vi "MOSES Background 4_v8.vi"(5 "Array Input":refnum<vi>) -> (0 "PSU":dbl[](graph), 1 "Values to Output":T1, 2 "Power Supply Filter Input":dbl[](graph), 3 "ROE":dbl[](graph))   [LabVIEW 2013]
uses:
  Instance           9 26Saved   MOSES Background 4 .vi
  Instance          14 26Saved   MOSES Background 4 .vi
  Instance           8 26Saved   MOSES Background 4 .vi
  Instance          21 26Saved   MOSES Background 4 .vi
  Instance           3 26Saved   MOSES Background 4 .vi
  Instance          22 26Saved   MOSES Background 4 .vi
  Instance           6 26Saved   MOSES Background 4 .vi
  Instance          23 26Saved   MOSES Background 4 .vi
  Instance           7 26Saved   MOSES Background 4 .vi
  Instance          24 26Saved   MOSES Background 4 .vi
  Instance           5 26Saved   MOSES Background 4 .vi
  Instance          15 26Saved   MOSES Background 4 .vi
  Instance           4 26Saved   MOSES Background 4 .vi
  Instance          16 26Saved   MOSES Background 4 .vi
  Instance          28 26Saved   MOSES Background 4 .vi
  Instance          17 26Saved   MOSES Background 4 .vi
  Instance           2 26Saved   MOSES Background 4 .vi
  Instance          18 26Saved   MOSES Background 4 .vi
  Instance           1 26Saved   MOSES Background 4 .vi
  Instance          19 26Saved   MOSES Background 4 .vi
  Instance          12 26Saved   MOSES Background 4 .vi
  Instance          20 26Saved   MOSES Background 4 .vi
  Instance          10 26Saved   MOSES Background 4 .vi
  Instance          26 26Saved   MOSES Background 4 .vi
  Instance          11 26Saved   MOSES Background 4 .vi
  Instance          25 26Saved   MOSES Background 4 .vi
  Instance          13 26Saved   MOSES Background 4 .vi
  Instance          27 26Saved   MOSES Background 4 .vi
panel:
  out "Boolean 17":bool
  out "Boolean 16":bool
  out "Boolean 15":bool
  out "Boolean 14":bool
  out "Boolean 13":bool
  out "Boolean 41":bool
  out "Boolean 40":bool
  out "Boolean 39":bool
  out "Boolean 38":bool
  out "Boolean 37":bool
  out "Boolean 36":bool
  out "Boolean 35":bool
  out "Boolean 34":bool
  out "Boolean 33":bool
  out "Boolean 32":bool
  out "Boolean 12":bool
  out "Boolean 11":bool
  out "Boolean 10":bool
  out "Boolean 84":bool
  out "Boolean 83":bool
  out "T_PSU, PSU Temp.":dbl
  out "Boolean 82":bool
  out "Boolean 81":bool
  out "T_ROE, ROE Temp.":dbl
  in  "stop 4":bool
  out "ROE_PSI, ROE power supply input current":dbl
  out "ROE_PSV, ROE power supply input voltage":dbl
  out "I_pf5, Premod filter 5V input current":dbl
  out "HAFI, H-alpha filter current":dbl
  out "S28I, Shutter 28V power current":dbl
  out "Ipf12+, Premod filter positive 12V input current":dbl
  out "If_in":dbl[](graph)
  out "Boolean 31":bool
  out "Boolean 30":bool
  out "Boolean 29":bool
  out "If_in, Power supply filter input current":dbl
  out "Boolean 23":bool
  out "Boolean 22":bool
  out "Boolean 9":bool
  out "Boolean 8":bool
  out "Boolean 7":bool
  out "HACV, H-alpha camera voltage":dbl
  out "HAFV, H-alpha filter voltage":dbl
  out "Boolean 21":bool
  out "Boolean 20":bool
  out "Boolean 19":bool
  out "Boolean 18":bool
  out "S28V, Shutter 28V power voltage":dbl
  out "T5V, Thermal 5V power voltage":dbl
  out "V5s, MGA2805S output voltage":dbl
  out "Vina_0y":dbl
  out "Vina_-y":dbl
  out "Vina_+y, INA330 Output":dbl
  out "Vex_0y":dbl
  out "Vex_-y":dbl
  out "Vex_+y":dbl
  out "Va_0y":dbl
  out "Va_-y":dbl
  out "Waveform Chart 2":dbl[](graph)
  out "Va_+y, Thermistor Voltage":dbl
  # "A"
  # "A"
  # "V"
  # "mA"
  # "C"
  # "C"
  # "V"
  # "V"
  # "V"
  # "V"
  # "V"
  # "A"
  # "mA"
  # "mA"
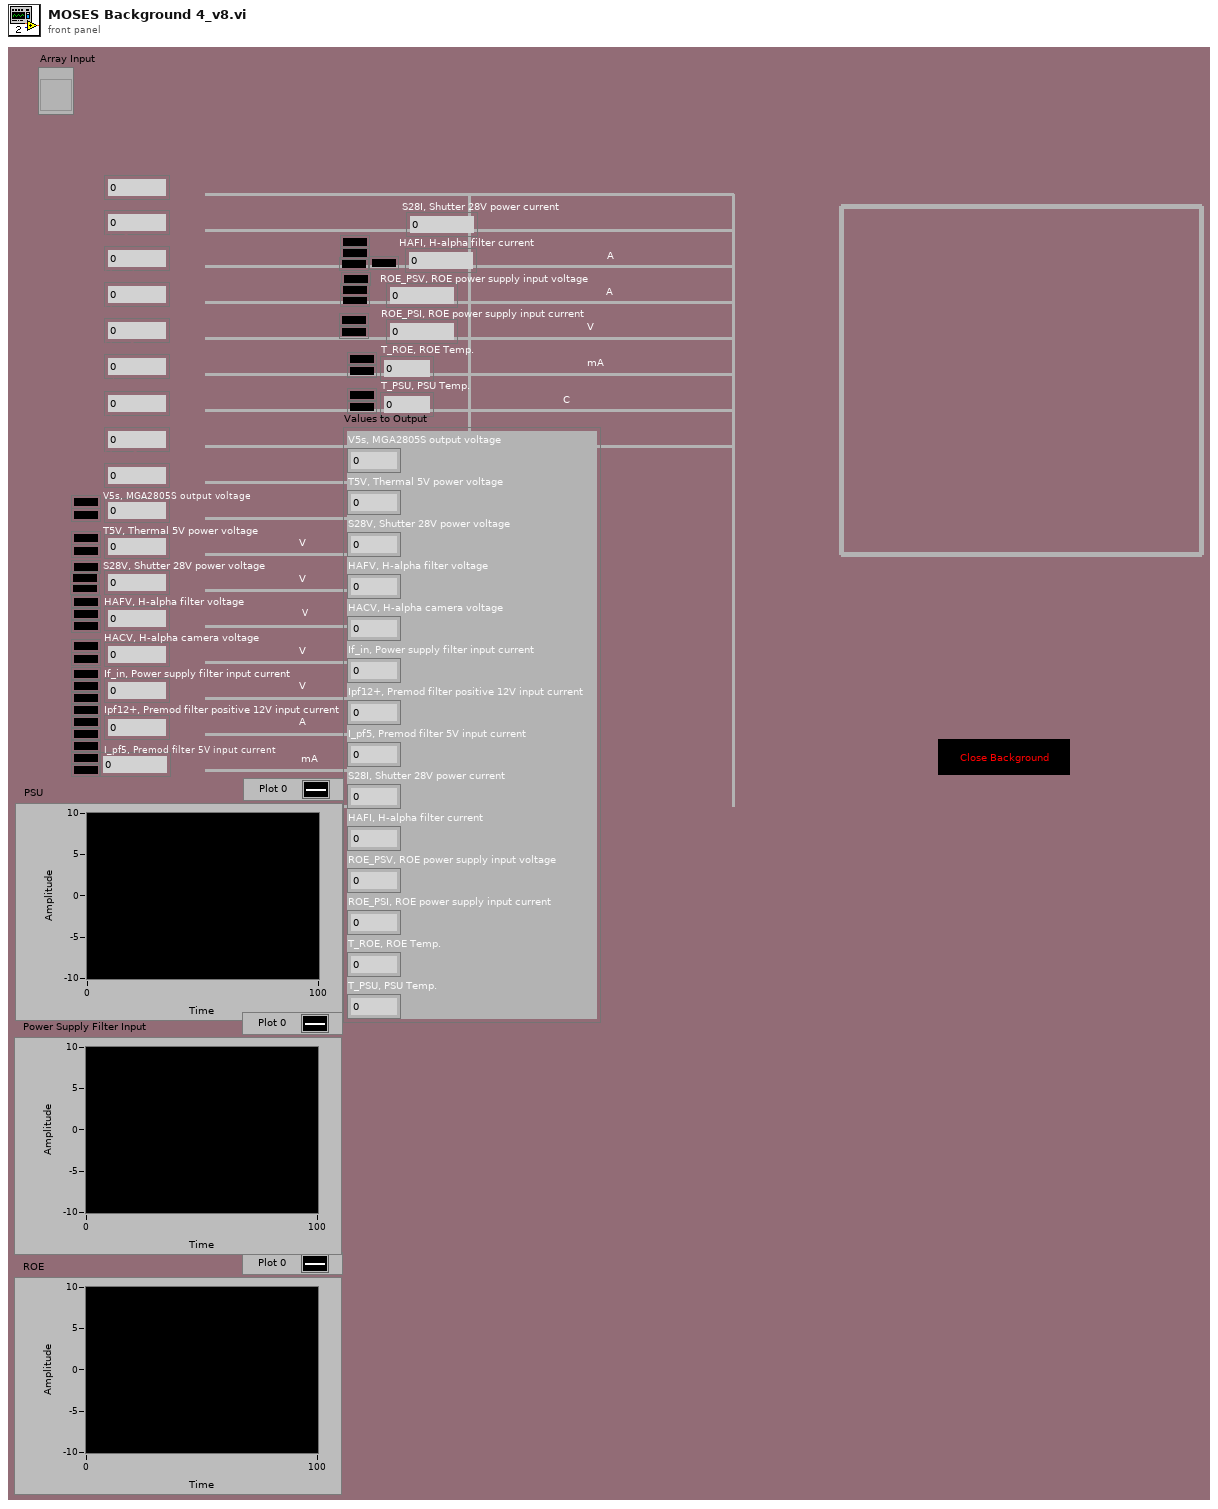
[diagram p1: front panel]
types:
  T1 = cluster{"V5s, MGA2805S output voltage":dbl, "T5V, Thermal 5V power voltage":dbl, "S28V, Shutter 28V power voltage":dbl, "HAFV, H-alpha filter voltage":dbl, "HACV, H-alpha camera voltage":dbl, "If_in, Power supply filter input current":dbl, "Ipf12+, Premod filter positive 12V input current":dbl, "I_pf5, Premod filter 5V input current":dbl, "S28I, Shutter 28V power current":dbl, "HAFI, H-alpha filter current":dbl, "ROE_PSV, ROE power supply input voltage":dbl, "ROE_PSI, ROE power supply input current":dbl, "T_ROE, ROE Temp.":dbl, "T_PSU, PSU Temp.":dbl}
  T2 = cluster{"Value[0]":dbl, "Value[1]":dbl, "Value[2]":dbl, "Value[3]":dbl, "Value[4]":dbl, "Value[5]":dbl, "Value[6]":dbl, "Value[7]":dbl, "Value[8]":dbl, "Value[9]":dbl, "Value[10]":dbl, "Value[11]":dbl, "Value[12]":dbl, "Value[13]":dbl, "Value[14]":dbl, "Value[15]":dbl, "Value[16]":dbl, "Value[17]":dbl, "Value[18]":dbl, "Value[19]":dbl, "Value[20]":dbl, "Value[21]":dbl, "Value[22]":dbl, "Value[23]":dbl, "Value[24]":dbl, "Value[25]":dbl, "Value[26]":dbl, "Value[27]":dbl, "Value[28]":dbl, "Value[29]":dbl, "Value[30]":dbl, "Value[31]":dbl, "Value[32]":dbl, "Value[33]":dbl, "Value[34]":dbl, "Value[35]":dbl, "Value[36]":dbl, "Value[37]":dbl, "Value[38]":dbl, "Value[39]":dbl, "Value[40]":dbl, "Value[41]":dbl, "Value[42]":dbl, "Value[43]":dbl, "Value[44]":dbl, "Value[45]":dbl, "Value[46]":dbl, "Value[47]":dbl, "Value[48]":dbl, "Value[49]":dbl, "Value[50]":dbl, "Value[51]":dbl, "Value[52]":dbl, "Value[53]":dbl, "Value[54]":dbl, "Value[55]":dbl, "Value[56]":dbl, "Value[57]":dbl, "Value[58]":dbl, "Value[59]":dbl, "Value[60]":dbl, "Value[61]":dbl, "Value[62]":dbl, "Value[63]":dbl, "Value[64]":dbl, "Value[65]":dbl, "Value[66]":dbl, "Value[67]":dbl, "Value[68]":dbl, "Value[69]":dbl}
  T3 = cluster{"[0]":dbl, "[1]":dbl, "[2]":dbl, "[3]":dbl, "[4]":dbl, "[5]":dbl, "[6]":dbl, "[7]":dbl, "[8]":dbl, "[9]":dbl, "[10]":dbl, "[11]":dbl, "[12]":dbl, "[13]":dbl}
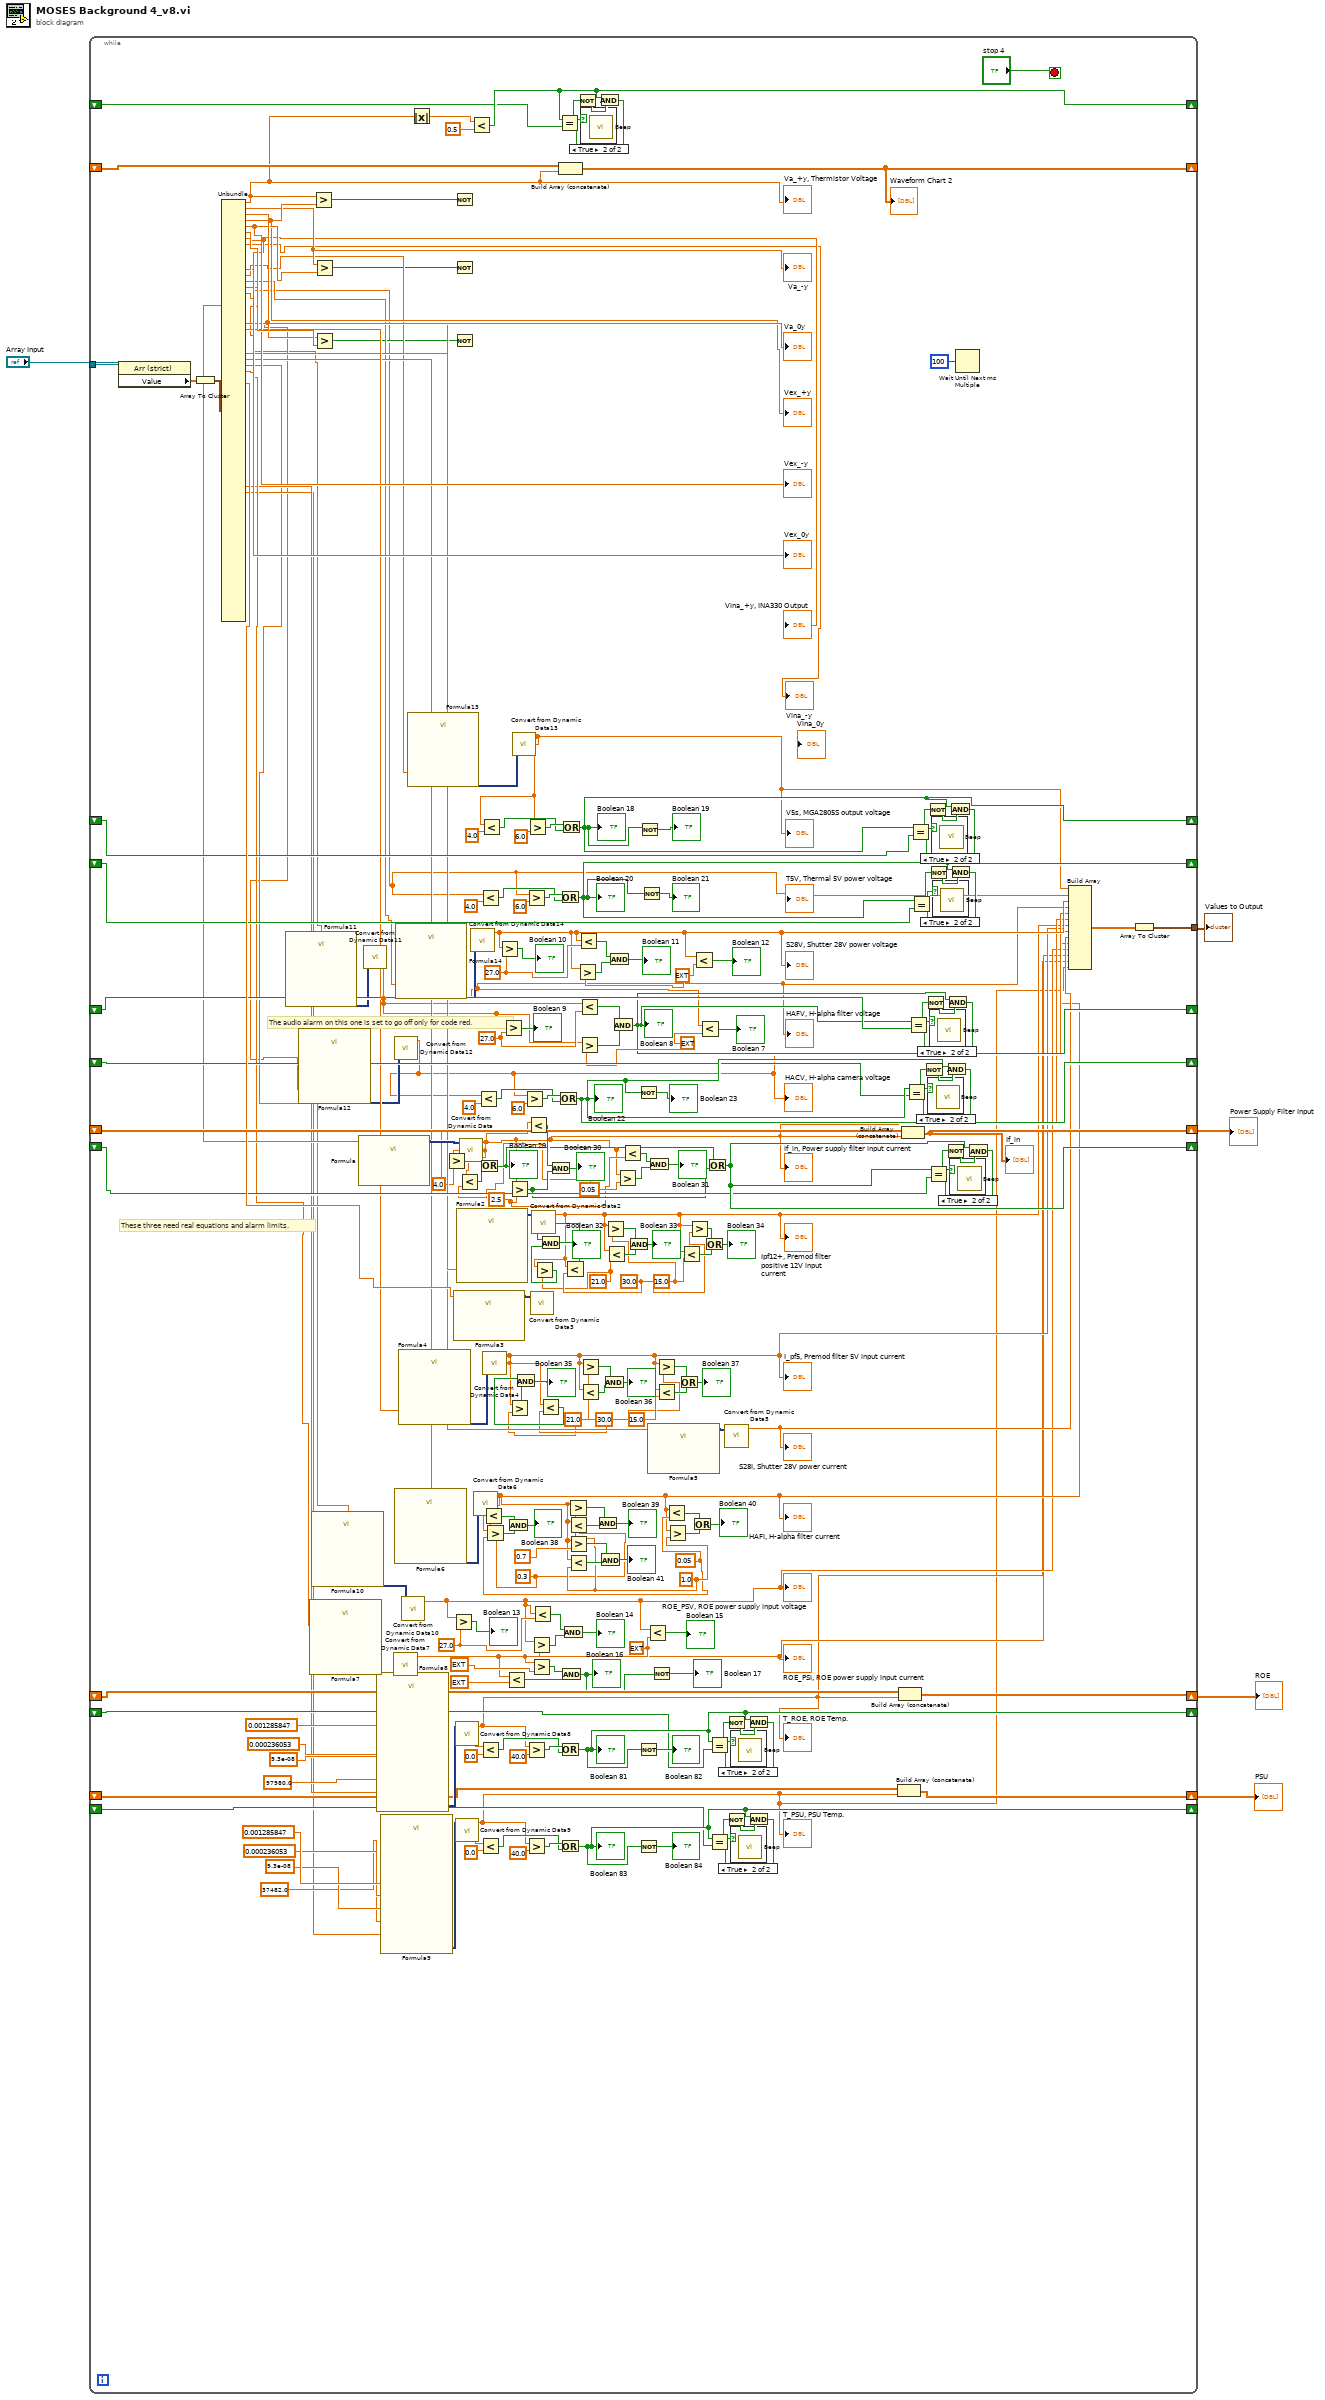
[diagram p0: block diagram]
diagram:
  n1 = while {
    tunnel: "Array Input" -> [w226]
    shift-right: [w222] -> _
    shift-left: _ -> [w223]
    shift-right: [w198] -> w1
    shift-left: _ -> [w199]
    shift-right: [w180] -> _
    shift-left: _ -> [w179]
    shift-right: [w163] -> _
    shift-left: _ -> [w162]
    shift-right: [w96] -> _
    shift-left: _ -> [w161]
    shift-right: [w160] -> _
    shift-left: _ -> [w159]
    shift-right: [w158] -> _
    shift-left: _ -> [w157]
    shift-right: [w156] -> _
    shift-left: _ -> [w155]
    shift-right: [w135] -> _
    shift-left: _ -> [w134]
    shift-right: [w133] -> _
    shift-left: _ -> [w132]
    shift-right: [w129] -> w3
    shift-left: _ -> [w131]
    shift-right: [w128] -> w2
    shift-left: _ -> [w130]
    tunnel: [w6] -> w4
    stop <- "stop 4" stop-if-true
    w42 = 27.0 ("y")
    w37 = ext 20.0 ("y")
    w45 = 0.05 ("y")
    w44 = 0.3 ("y")
    w46 = 1.0 ("y")
    w62 = 15.0 ("y")
    w61 = 30.0 ("y")
    w60 = 21.0 ("y")
    w73 = 15.0 ("y")
    w72 = 30.0 ("y")
    w22 = 21.0 ("y")
    w94 = 27.0 ("y")
    w90 = ext 20.0 ("y")
    w27 = 0.05 ("y")
    w85 = 4.0 ("y")
    w23 = 2.5 ("y")
    w99 = ext 20.0 ("y")
    w206 = 27.0 ("y")
    # "These three need real equations and alarm limits."
    # "The audio alarm on this one is set to go off only for code red."
    n2 = property class="Arr (strict)"(reference=w226) -> ("Value"=w225:dbl[])  [unwired: 1 in, 2 out]
    n3 = Array To Cluster(array=w225) -> (cluster=w224:T2)
    n4 = Unbundle(w224) -> ("Value[0]"=w186:dbl, "Value[1]"=w187:dbl, "Value[2]"=w220:dbl, "Value[3]"=w188:dbl, "Value[4]"=w219:dbl, "Value[5]"=w221:dbl, "Value[6]"=→"Vex_0y" →"Vina_+y, INA330 Output":dbl, "Value[7]"=→"Vina_-y":dbl, "Value[11]"=w102:dbl, "Value[12]"=w20:dbl, "Value[13]"=w100:dbl, "Value[14]"=w104:dbl, "Value[15]"=w106:dbl, "Value[17]"=w125:dbl, "Value[20]"=w124:dbl, "Value[21]"=w123:dbl, "Value[25]"=w122:dbl, "Value[26]"=w121:dbl, "Value[27]"=w108:dbl, "Value[28]"=w120:dbl, "Value[30]"=w195:dbl, "Value[47]"=w111:dbl, "Value[48]"=w110:dbl)  [unwired: 47 out]
    "Va_+y, Thermistor Voltage" <- w186
    "Va_-y" <- w187
    "Va_0y" <- w220
    "Vex_+y" <- w188
    "Vex_-y" <- w219
    "T5V, Thermal 5V power voltage" <- w20
    n5 = call "Formula11"("X1"=w104) -> ("Result"=w105:dynamicdata)  [unwired: 13 in, 1 out]
    n6 = call "Formula12"("X1"=w106) -> ("Result"=w107:dynamicdata)  [unwired: 13 in, 1 out]
    n7 = call "Formula7"("X1"=w120) -> ("Result"=w191:dynamicdata)  [unwired: 13 in, 1 out]
    n8 = Greater?(x=w186, y=w188) -> (0:w190:bool)
    n9 = call "Formula10"("X1"=w108) -> ("Result"=w109:dynamicdata)  [unwired: 13 in, 1 out]
    n10 = Greater?(x=w187, y=w219) -> (0:w84:bool)
    n11 = Greater?(x=w220, y=w221) -> (0:w83:bool)
    n12 = call "Formula"("X1"=w125) -> ("Result"=w200:dynamicdata)  [unwired: 13 in, 1 out]
    n13 = call "Convert from Dynamic Data11"("Dynamic Data Type"=w105) -> ("Scalar"=w18:dbl)  [unwired: 3 in]
    "HAFV, H-alpha filter voltage" <- w18
    n14 = call "Formula8"("a"=0.001285847 ("double precision float"), "v0"=w111, "b"=0.000236053 ("double precision float"), "c"=9.3e-08 ("double precision float"), "R"=97980.0 ("double precision float")) -> ("Result"=w148:dynamicdata)  [unwired: 9 in, 1 out]
    n15 = call "Formula9"("a"=0.001285847 ("double precision float"), "v0"=w110, "b"=0.000236053 ("double precision float"), "c"=9.3e-08 ("double precision float"), "R"=37482.0 ("double precision float")) -> ("Result"=w139:dynamicdata)  [unwired: 9 in, 1 out]
    n16 = call "Convert from Dynamic Data7"("Dynamic Data Type"=w191) -> ("Scalar"=w10:dbl)  [unwired: 3 in]
    "ROE_PSI, ROE power supply input current" <- w10
    n17 = call "Convert from Dynamic Data12"("Dynamic Data Type"=w107) -> ("Scalar"=w17:dbl)  [unwired: 3 in]
    "HACV, H-alpha camera voltage" <- w17
    n18 = call "Formula6"("X1"=w121) -> ("Result"=w192:dynamicdata)  [unwired: 13 in, 1 out]
    n19 = call "Formula14"("X1"=w100) -> ("Result"=w101:dynamicdata)  [unwired: 13 in, 1 out]
    n20 = call "Formula4"("X1"=w123) -> ("Result"=w194:dynamicdata)  [unwired: 13 in, 1 out]
    n21 = call "Convert from Dynamic Data10"("Dynamic Data Type"=w109) -> ("Scalar"=w11:dbl)  [unwired: 3 in]
    "ROE_PSV, ROE power supply input voltage" <- w11
    n22 = call "Formula13"("X1"=w102) -> ("Result"=w103:dynamicdata)  [unwired: 13 in, 1 out]
    n23 = Absolute Value(x=w186) -> (abs(x)=w184:dbl)
    n24 = Greater?(x=w11, y=w42) -> (0:→"Boolean 13":bool)
    n25 = Not(x=w190) -> ()  [unwired: 1 out]
    n26 = Not(x=w84) -> ()  [unwired: 1 out]
    n27 = Not(x=w83) -> ()  [unwired: 1 out]
    n28 = call "Formula3"("X1"=w195) -> ("Result"=w196:dynamicdata)  [unwired: 13 in, 1 out]
    n29 = call "Convert from Dynamic Data8"("Dynamic Data Type"=w148) -> ("Scalar"=w9:dbl)  [unwired: 3 in]
    "T_ROE, ROE Temp." <- w9
    n30 = call "Convert from Dynamic Data9"("Dynamic Data Type"=w139) -> ("Scalar"=w8:dbl)  [unwired: 3 in]
    "T_PSU, PSU Temp." <- w8
    n31 = call "Formula2"("X1"=w124) -> ("Result"=w197:dynamicdata)  [unwired: 13 in, 1 out]
    n32 = call "Convert from Dynamic Data"("Dynamic Data Type"=w200) -> ("Scalar"=w16:dbl)  [unwired: 3 in]
    "If_in, Power supply filter input current" <- w16
    n33 = Greater?(x=w16, y=w85) -> (0:w28:bool)
    n34 = Less?(x=w16, y=w27) -> (x < y?=w30:bool)
    n35 = Less?(x=w184, y=0.5) -> (x < y?=w180:bool)
    n36 = call "Convert from Dynamic Data14"("Dynamic Data Type"=w101) -> ("Scalar"=w19:dbl)  [unwired: 3 in]
    "S28V, Shutter 28V power voltage" <- w19
    n37 = call "Convert from Dynamic Data6"("Dynamic Data Type"=w192) -> ("Scalar"=w12:dbl)  [unwired: 3 in]
    "HAFI, H-alpha filter current" <- w12
    n38 = Less?(x=w17, y=4.0) -> (x < y?=w202:bool)
    n39 = Or(x=w28, y=w30) -> (x .or. y?=w29:bool)
    "Boolean 29" <- w29
    n40 = Less?(x=w20, y=4.0) -> (x < y?=w210:bool)
    n41 = Less?(x=w9, y=0.0) -> (x < y?=w150:bool)
    n42 = Less?(x=w8, y=0.0) -> (x < y?=w141:bool)
    n43 = Less?(x=w12, y=w44) -> (x < y?=w58:bool)
    n44 = call "Convert from Dynamic Data4"("Dynamic Data Type"=w194) -> ("Scalar"=w14:dbl)  [unwired: 3 in]
    "I_pf5, Premod filter 5V input current" <- w14
    n45 = Greater?(x=w12, y=w45) -> (0:w59:bool)
    n46 = Greater?(x=w19, y=w94) -> (0:→"Boolean 10":bool)
    n47 = Greater?(x=w18, y=w206) -> (0:→"Boolean 9":bool)
    n48 = Less?(x=w10, y=ext 390.0) -> (x < y?=w34:bool)
    n49 = And(x=w58, y=w59) -> (x .and. y?=→"Boolean 38":bool)
    n50 = Greater?(x=w16, y=w23) -> (0:w88:bool)
    n51 = Greater?(x=w14, y=w60) -> (0:w71:bool)
    n52 = call "Convert from Dynamic Data13"("Dynamic Data Type"=w103) -> ("Scalar"=w21:dbl)  [unwired: 3 in]
    "V5s, MGA2805S output voltage" <- w21
    n53 = Less?(x=w21, y=4.0) -> (x < y?=w215:bool)
    n54 = Greater?(x=w17, y=6.0) -> (0:w203:bool)
    n55 = Greater?(x=w20, y=6.0) -> (0:w211:bool)
    n56 = Greater?(x=w9, y=40.0) -> (0:w151:bool)
    n57 = Greater?(x=w8, y=40.0) -> (0:w142:bool)
    n58 = Greater?(x=w21, y=6.0) -> (0:w216:bool)
    n59 = Less?(x=w16, y=w85) -> (x < y?=w86:bool)
    n60 = Greater?(x=w10, y=ext 250.0) -> (0:w33:bool)
    n61 = call "Convert from Dynamic Data3"("Dynamic Data Type"=w196) -> ()  [unwired: 3 in, 1 out]
    n62 = Greater?(x=w11, y=w37) -> (0:w41:bool)
    n63 = Less?(x=w11, y=w42) -> (x < y?=w40:bool)
    n64 = call "Convert from Dynamic Data2"("Dynamic Data Type"=w197) -> ("Scalar"=w15:dbl)  [unwired: 3 in]
    "Ipf12+, Premod filter positive 12V input current" <- w15
    n65 = Greater?(x=w15, y=w22) -> (0:w82:bool)
    n66 = Less?(x=w14, y=w61) -> (x < y?=w70:bool)
    n67 = And(x=w70, y=w71) -> (x .and. y?=→"Boolean 35":bool)
    n68 = And(x=w86, y=w88) -> (x .and. y?=→"Boolean 30":bool)
    n69 = Or(x=w203, y=w202) -> (x .or. y?=w163:bool)
    "Boolean 22" <- w163
    n70 = Equal?(x=w180, y=w179) -> (x = y?=w181:bool)
    n71 = Build Array (concatenate)(w223, w186) -> (w222:dbl[])
    "Waveform Chart 2" <- w222
    n72 = Or(x=w211, y=w210) -> (x .or. y?=w160:bool)
    "Boolean 20" <- w160
    n73 = Or(x=w151, y=w150) -> (x .or. y?=w135:bool)
    "Boolean 81" <- w135
    n74 = Or(x=w142, y=w141) -> (x .or. y?=w133:bool)
    "Boolean 83" <- w133
    n75 = Or(x=w216, y=w215) -> (x .or. y?=w158:bool)
    "Boolean 18" <- w158
    n76 = And(x=w33, y=w34) -> (x .and. y?=w32:bool)
    "Boolean 16" <- w32
    n77 = And(x=w40, y=w41) -> (x .and. y?=→"Boolean 14":bool)
    n78 = Less?(x=w15, y=w72) -> (x < y?=w81:bool)
    n79 = And(x=w81, y=w82) -> (x .and. y?=→"Boolean 32":bool)
    n80 = Greater?(x=w12, y=w44) -> (0:w56:bool)
    n81 = Less?(x=w12, y=w46) -> (x < y?=w55:bool)
    n82 = Greater?(x=w12, y=0.7) -> (0:w52:bool)
    n83 = Less?(x=w12, y=w46) -> (x < y?=w53:bool)
    n84 = Not(x=w181) -> (.not. x?=w182:bool)
    n85 = Greater?(x=w19, y=w90) -> (0:w93:bool)
    n86 = Less?(x=w19, y=w94) -> (x < y?=w92:bool)
    n87 = Less?(x=w18, y=w206) -> (x < y?=w98:bool)
    n88 = Greater?(x=w18, y=w99) -> (0:w97:bool)
    n89 = Greater?(x=w14, y=w62) -> (0:w67:bool)
    n90 = Less?(x=w14, y=w60) -> (x < y?=w68:bool)
    n91 = And(x=w56, y=w55) -> (x .and. y?=→"Boolean 39":bool)
    n92 = And(x=w180, y=w182) -> (x .and. y?=w183:bool)
    n93 = case shown="True" w183 {
      frame False {
      }
      frame True {
        n94 = call <vilib>:"Beep.vi"() -> ()  [unwired: 12 in]
      }
    }
    n95 = And(x=w52, y=w53) -> (x .and. y?=→"Boolean 41":bool)
    n96 = And(x=w67, y=w68) -> (x .and. y?=→"Boolean 36":bool)
    n97 = Greater?(x=w15, y=w73) -> (0:w78:bool)
    n98 = Less?(x=w15, y=w22) -> (x < y?=w77:bool)
    n99 = And(x=w92, y=w93) -> (x .and. y?=→"Boolean 11":bool)
    n100 = And(x=w98, y=w97) -> (x .and. y?=w96:bool)
    "Boolean 8" <- w96
    n101 = Greater?(x=w16, y=w27) -> (0:w26:bool)
    n102 = Less?(x=w16, y=w23) -> (x < y?=w24:bool)
    n103 = And(x=w78, y=w77) -> (x .and. y?=→"Boolean 33":bool)
    n104 = Not(x=w163) -> (.not. x?=→"Boolean 23":bool)
    n105 = Not(x=w135) -> (.not. x?=→"Boolean 82":bool)
    n106 = Not(x=w133) -> (.not. x?=→"Boolean 84":bool)
    n107 = Not(x=w158) -> (.not. x?=→"Boolean 19":bool)
    n108 = Not(x=w160) -> (.not. x?=→"Boolean 21":bool)
    n109 = Less?(x=w11, y=w37) -> (x < y?=→"Boolean 15":bool)
    n110 = And(x=w24, y=w26) -> (x .and. y?=→"Boolean 31":bool)
    n111 = call "Formula5"("X1"=w122) -> ("Result"=w193:dynamicdata)  [unwired: 13 in, 1 out]
    n112 = Not(x=w32) -> (.not. x?=→"Boolean 17":bool)
    n113 = Greater?(x=w14, y=w61) -> (0:w64:bool)
    n114 = Less?(x=w14, y=w62) -> (x < y?=w65:bool)
    n115 = Less?(x=w12, y=w45) -> (x < y?=w49:bool)
    n116 = Greater?(x=w12, y=w46) -> (0:w50:bool)
    n117 = Or(x=w64, y=w65) -> (x .or. y?=→"Boolean 37":bool)
    n118 = Less?(x=w15, y=w73) -> (x < y?=w75:bool)
    n119 = Greater?(x=w15, y=w72) -> (0:w74:bool)
    n120 = Or(x=w49, y=w50) -> (x .or. y?=→"Boolean 40":bool)
    n121 = Less?(x=w19, y=w90) -> (x < y?=→"Boolean 12":bool)
    n122 = Less?(x=w18, y=w99) -> (x < y?=→"Boolean 7":bool)
    n123 = Or(x=w74, y=w75) -> (x .or. y?=→"Boolean 34":bool)
    n124 = Or(x=w29, y=w88) -> (x .or. y?=w156:bool)
    n125 = Equal?(x=w135, y=w134) -> (x = y?=w145:bool)
    n126 = Equal?(x=w133, y=w132) -> (x = y?=w136:bool)
    n127 = call "Convert from Dynamic Data5"("Dynamic Data Type"=w193) -> ("Scalar"=w13:dbl)  [unwired: 3 in]
    "S28I, Shutter 28V power current" <- w13
    n128 = Not(x=w145) -> (.not. x?=w146:bool)
    n129 = Not(x=w136) -> (.not. x?=w137:bool)
    n130 = And(x=w135, y=w146) -> (x .and. y?=w147:bool)
    n131 = case shown="True" w147 {
      frame False {
      }
      frame True {
        n132 = call <vilib>:"Beep.vi"() -> ()  [unwired: 12 in]
      }
    }
    n133 = And(x=w133, y=w137) -> (x .and. y?=w138:bool)
    n134 = case shown="True" w138 {
      frame False {
      }
      frame True {
        n135 = call <vilib>:"Beep.vi"() -> ()  [unwired: 12 in]
      }
    }
    n136 = Build Array (concatenate)(w130, w8) -> (w128:dbl[])
    n137 = Build Array (concatenate)(w131, w9) -> (w129:dbl[])
    n138 = Build Array (concatenate)(w199, w16) -> (w198:dbl[])
    "If_in" <- w198
    n139 = Equal?(x=w163, y=w162) -> (x = y?=w167:bool)
    n140 = Equal?(x=w96, y=w161) -> (x = y?=w170:bool)
    n141 = Equal?(x=w158, y=w157) -> (x = y?=w176:bool)
    n142 = Equal?(x=w160, y=w159) -> (x = y?=w173:bool)
    n143 = Not(x=w167) -> (.not. x?=w168:bool)
    n144 = Not(x=w170) -> (.not. x?=w171:bool)
    n145 = Not(x=w176) -> (.not. x?=w177:bool)
    n146 = Not(x=w173) -> (.not. x?=w174:bool)
    n147 = Equal?(x=w156, y=w155) -> (x = y?=w164:bool)
    n148 = Not(x=w164) -> (.not. x?=w165:bool)
    n149 = And(x=w163, y=w168) -> (x .and. y?=w169:bool)
    n150 = case shown="True" w169 {
      frame False {
      }
      frame True {
        n151 = call <vilib>:"Beep.vi"() -> ()  [unwired: 12 in]
      }
    }
    n152 = And(x=w96, y=w171) -> (x .and. y?=w172:bool)
    n153 = case shown="True" w172 {
      frame False {
      }
      frame True {
        n154 = call <vilib>:"Beep.vi"() -> ()  [unwired: 12 in]
      }
    }
    n155 = And(x=w158, y=w177) -> (x .and. y?=w178:bool)
    n156 = case shown="True" w178 {
      frame False {
      }
      frame True {
        n157 = call <vilib>:"Beep.vi"() -> ()  [unwired: 12 in]
      }
    }
    n158 = And(x=w160, y=w174) -> (x .and. y?=w175:bool)
    n159 = case shown="True" w175 {
      frame False {
      }
      frame True {
        n160 = call <vilib>:"Beep.vi"() -> ()  [unwired: 12 in]
      }
    }
    n161 = Wait Until Next ms Multiple(millisecond multiple=u32 100) -> ()  [unwired: 1 out]
    n162 = And(x=w156, y=w165) -> (x .and. y?=w166:bool)
    n163 = case shown="True" w166 {
      frame False {
      }
      frame True {
        n164 = call <vilib>:"Beep.vi"() -> ()  [unwired: 12 in]
      }
    }
    n165 = Build Array(w21, w20, w19, w18, w17, w16, w15, w14, w13, w12, w11, w10, w9, w8) -> (w7:dbl[])
    n166 = Array To Cluster(array=w7) -> (cluster=w6:T3)
  }
  "Values to Output" <- w4
  "ROE" <- w3
  "PSU" <- w2
  "Power Supply Filter Input" <- w1
